vi "Init Dashboard Panel.vi"(8 "error in (no error)":errorcluster, 11 "SB App in":refnum<class "SB App.lvclass">) -> (0 "error out":errorcluster, 3 "SB App out":refnum<class "SB App.lvclass">)   [LabVIEW 2020, in "SB App.lvlib" / "SB App.lvclass"]
uses:
  SB App.lvclass
  Dashboard Panel/Dashboard Panel.lvclass
  C:/Program Files (x86)/National Instruments/LabVIEW 2020/vi.lib/IlluminatedG/IG OOPanel/OOPanel/Panel/Panel.lvclass
  SB App.lvclass/SB App.ctl
  <vilib>/IlluminatedG/IG OOPanel/OOPanel/Manager/Manager.lvclass
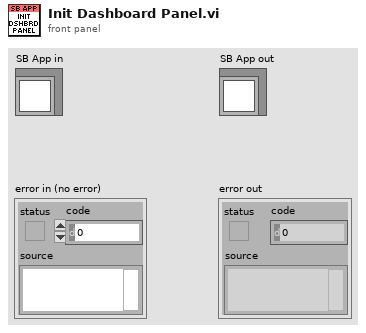
[diagram p1: front panel]
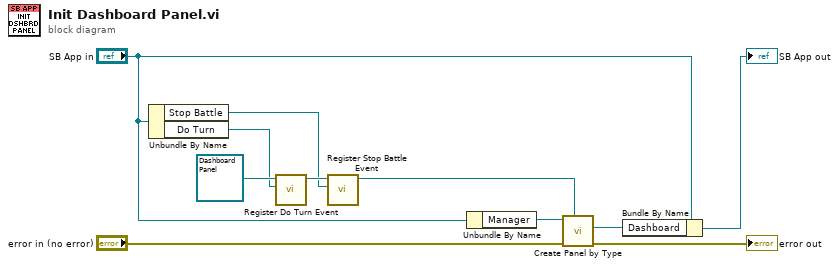
[diagram p0: block diagram]
diagram:
  n1 = Unbundle By Name("SB App in") -> ("Stop Battle"=w1:refnum<user-event>, "Do Turn"=w7:refnum<user-event>)
  n2 = call "Register Do Turn Event.vi"("Do Turn"=w7, "Dashboard Panel in"=refnum<class "Dashboard Panel.lvclass"> refnum ("SB App.lvlib:Dashboard Panel.lvclass")) -> ("Dashboard Panel out"=w3:refnum<class "Dashboard Panel.lvclass">)  [unwired: 8 in, 1 out]
  n3 = call "Register Stop Battle Event.vi"("Stop Battle"=w1, "Dashboard Panel in"=w3) -> ("Dashboard Panel out"=w2:refnum<class "Dashboard Panel.lvclass">)  [unwired: 8 in, 1 out]
  n4 = Unbundle By Name("SB App in") -> ("Manager"=w11:refnum<class "Manager.lvclass">)
  n5 = call <vilib>:"Create Panel by Type.vi"("Panel Type"=w2, "error in (no error)"="error in (no error)", "Manager in"=w11) -> ("error out"=→"error out":errorcluster, "Panel"=w5:refnum<class "Dashboard Panel.lvclass">)  [unwired: 6 in, 1 out]
  n6 = Bundle By Name(cluster="SB App in", "Dashboard"=w5) -> (→"SB App out":refnum<class "SB App.lvclass">)
